vi "GE 5565PIORC.Memory.In-Place Read from DMA Block.vi"   [LabVIEW 2016, in "GE 5565PIORC.lvclass"]
doc: "Reads <B>count</B> elements from the provided <B>Block Descriptor</B> into the provided <B>data</B> array. The number of elements transferred will be either <B>count</B> or the number of elements in <B>data</B>, whichever is smaller."
uses:
  GE 5565PIORC.lvclass
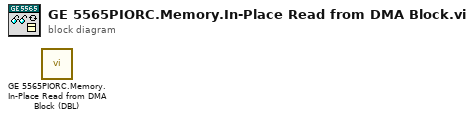
[diagram p0: block diagram]
diagram:
  n1 = call "GE 5565PIORC.Memory.In-Place Read from DMA Block (DBL).vi"() -> ()  [unwired: 8 in, 4 out]
